vi "Get Test Info.vi"(7 "error in (no error)":errorcluster, 10 "Sequence Context In":T1) -> (0 "error out":errorcluster, 2 "Test Results":string[][](array[string]), 3 "Sequence Context out":T1)   [LabVIEW 2010]
uses:
  <vilib>/addons/TestStand/_TSLegacy.llb/LabVIEW Test - Sequence Context.ctl
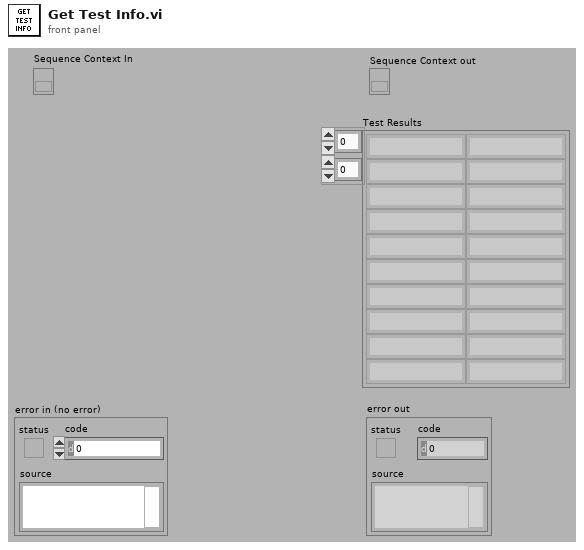
[diagram p1: front panel]
types:
  T1 = typedef "LabVIEW Test - Sequence Context.ctl" = refnum<k7>
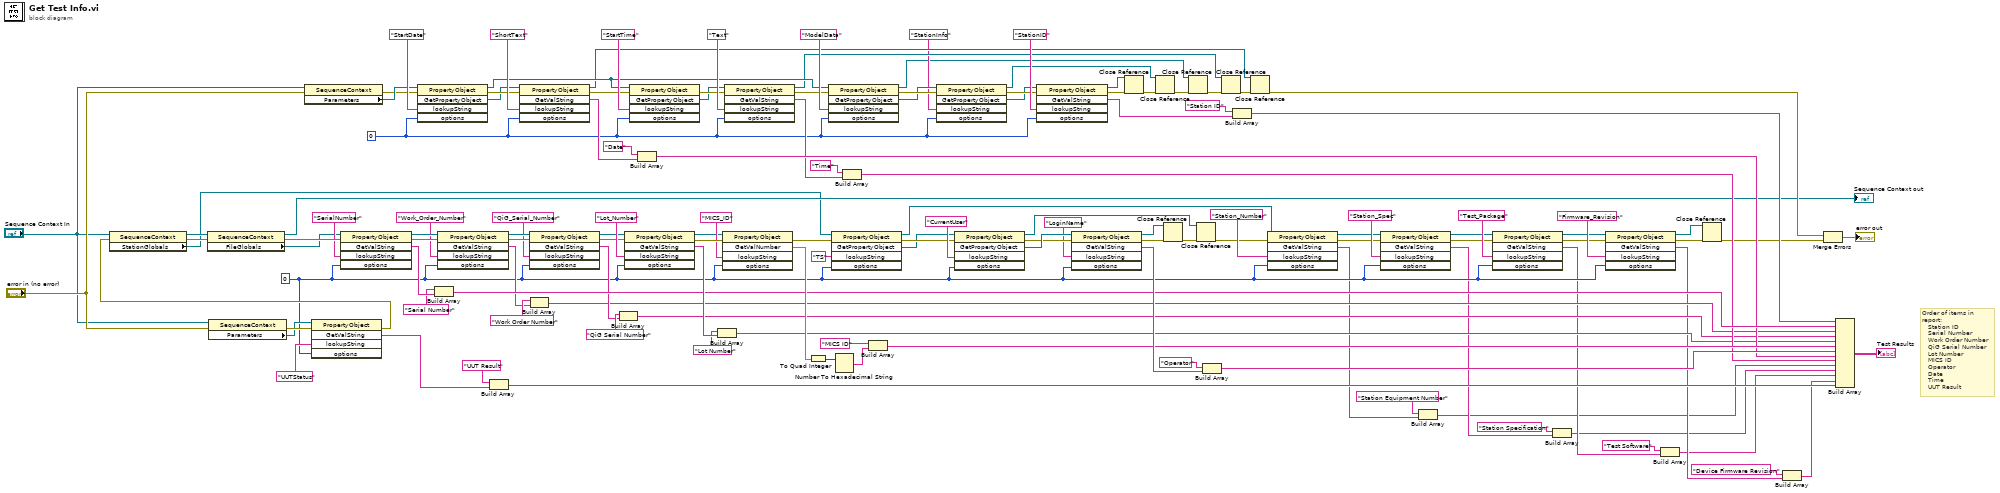
[diagram p0: block diagram]
diagram:
  w65 = 0
  w18 = 0
  # "Order of items in report:\n   Station ID\n   Serial Number\n   Work Order Number\n   QiG Serial Number\n   Lot Number\n   MICS ID\n   Operator\n   Date\n   Time\n   UUT Result"
  n1 = property class="SequenceContext"(reference="Sequence Context In", error in="error in (no error)") -> (error out=w37:errorcluster, "Parameters"=w36:refnum<k7>)  [unwired: 1 out]
  n2 = property class="SequenceContext"(reference="Sequence Context In", error in="error in (no error)") -> (error out=w95:errorcluster, "Parameters"=w100:refnum<k7>)  [unwired: 1 out]
  n3 = invoke class="PropertyObject" method="GetValString"(reference=w36, error in=w37, "lookupString"="UUTStatus", "options"=w18) -> (error out=w35:errorcluster, "GetValString"=w38:string)  [unwired: 1 in, 3 out]
  n4 = property class="SequenceContext"(reference="Sequence Context In", error in=w35) -> (reference out=w32:T1, error out=w34:errorcluster, "StationGlobals"=w31:refnum<k7>)
  n5 = property class="SequenceContext"(reference=w32, error in=w34) -> (reference out=→"Sequence Context out":T1, error out=w130:errorcluster, "FileGlobals"=w94:refnum<k7>)
  n6 = invoke class="PropertyObject" method="GetValString"(reference=w94, error in=w130, "lookupString"="SerialNumber", "options"=w18) -> (reference out=w55:refnum<k7>, error out=w54:errorcluster, "GetValString"=w124:string)  [unwired: 1 in, 2 out]
  n7 = invoke class="PropertyObject" method="GetPropertyObject"(reference=w100, error in=w95, "lookupString"="StartDate", "options"=w65) -> (reference out=w89:refnum<k7>, error out=w96:errorcluster, "GetPropertyObject"=w92:refnum<k7>)  [unwired: 1 in, 2 out]
  n8 = Build Array("Serial Number", w124) -> (w79:string[])
  n9 = invoke class="PropertyObject" method="GetValString"(reference=w55, error in=w54, "lookupString"="Work_Order_Number", "options"=w18) -> (reference out=w50:refnum<k7>, error out=w52:errorcluster, "GetValString"=w47:string)  [unwired: 1 in, 2 out]
  n10 = Build Array("UUT Result", w38) -> (w28:string[])
  n11 = invoke class="PropertyObject" method="GetValString"(reference=w92, error in=w96, "lookupString"="ShortText", "options"=w65) -> (reference out=w84:refnum<k7>, error out=w90:errorcluster, "GetValString"=w72:string)  [unwired: 1 in, 2 out]
  n12 = invoke class="PropertyObject" method="GetValString"(reference=w50, error in=w52, "lookupString"="QiG_Serial_Number", "options"=w18) -> (reference out=w46:refnum<k7>, error out=w51:errorcluster, "GetValString"=w44:string)  [unwired: 1 in, 2 out]
  n13 = Build Array("Work Order Number", w47) -> (w41:string[])
  n14 = Build Array("QiG Serial Number" ("lookupString"), w44) -> (w40:string[])
  n15 = invoke class="PropertyObject" method="GetValString"(reference=w46, error in=w51, "lookupString"="Lot_Number", "options"=w18) -> (reference out=w93:refnum<k7>, error out=w117:errorcluster, "GetValString"=w122:string)  [unwired: 1 in, 2 out]
  n16 = invoke class="PropertyObject" method="GetPropertyObject"(reference=w89, error in=w90, "lookupString"="StartTime", "options"=w65) -> (error out=w98:errorcluster, "GetPropertyObject"=w91:refnum<k7>)  [unwired: 1 in, 3 out]
  n17 = Build Array("Date" ("lookupString"), w72) -> (w74:string[])
  n18 = Build Array("Lot Number" ("lookupString"), w122) -> (w42:string[])
  n19 = invoke class="PropertyObject" method="GetValNumber"(reference=w93, error in=w117, "lookupString"="MICS_ID", "options"=w18) -> (error out=w115:errorcluster, "GetValNumber"=w112:dbl)  [unwired: 1 in, 3 out]
  n20 = invoke class="PropertyObject" method="GetValString"(reference=w91, error in=w98, "lookupString"="Text", "options"=w65) -> (reference out=w83:refnum<k7>, error out=w88:errorcluster, "GetValString"=w71:string)  [unwired: 1 in, 2 out]
  n21 = To Quad Integer(1:w112) -> (0:w113:i64)
  n22 = invoke class="PropertyObject" method="GetPropertyObject"(reference=w89, error in=w88, "lookupString"="ModelData", "options"=w65) -> (reference out=w62:refnum<k7>, error out=w69:errorcluster, "GetPropertyObject"=w67:refnum<k7>)  [unwired: 1 in, 2 out]
  n23 = invoke class="PropertyObject" method="GetPropertyObject"(reference=w31, error in=w115, "lookupString"="TS", "options"=w18) -> (reference out=w5:refnum<k7>, error out=w128:errorcluster, "GetPropertyObject"=w30:refnum<k7>)  [unwired: 1 in, 2 out]
  n24 = Number To Hexadecimal String(2:w113) -> (0:w114:string)  [unwired: 1 in]
  n25 = Build Array("Time" ("lookupString"), w71) -> (w73:string[])
  n26 = Build Array("MICS ID" ("lookupString"), w114) -> (w78:string[])
  n27 = invoke class="PropertyObject" method="GetPropertyObject"(reference=w67, error in=w69, "lookupString"="StationInfo", "options"=w65) -> (reference out=w57:refnum<k7>, error out=w68:errorcluster, "GetPropertyObject"=w64:refnum<k7>)  [unwired: 1 in, 2 out]
  n28 = invoke class="PropertyObject" method="GetPropertyObject"(reference=w30, error in=w128, "lookupString"="CurrentUser", "options"=w18) -> (reference out=w43:refnum<k7>, error out=w126:errorcluster, "GetPropertyObject"=w127:refnum<k7>)  [unwired: 1 in, 2 out]
  n29 = invoke class="PropertyObject" method="GetValString"(reference=w64, error in=w68, "lookupString"="StationID", "options"=w65) -> (reference out=w60:refnum<k7>, error out=w61:errorcluster, "GetValString"=w63:string)  [unwired: 1 in, 2 out]
  n30 = invoke class="PropertyObject" method="GetValString"(reference=w127, error in=w126, "lookupString"="LoginName", "options"=w18) -> (reference out=w106:refnum<k7>, error out=w107:errorcluster, "GetValString"=w120:string)  [unwired: 1 in, 2 out]
  n31 = Close Reference(reference=w60, error in (no error)=w61) -> (error out=w59:errorcluster)
  n32 = Close Reference(reference=w57, error in (no error)=w59) -> (error out=w58:errorcluster)
  n33 = Close Reference(reference=w106, error in (no error)=w107) -> (error out=w105:errorcluster)
  n34 = Close Reference(reference=w62, error in (no error)=w58) -> (error out=w87:errorcluster)
  n35 = Close Reference(reference=w43, error in (no error)=w105) -> (error out=w23:errorcluster)
  n36 = Build Array("Operator" ("lookupString"), w120) -> (w77:string[])
  n37 = Close Reference(reference=w83, error in (no error)=w87) -> (error out=w86:errorcluster)
  n38 = Build Array("Station ID" ("lookupString"), w63) -> (w80:string[])
  n39 = Close Reference(reference=w84, error in (no error)=w86) -> (error out=w85:errorcluster)
  n40 = invoke class="PropertyObject" method="GetValString"(reference=w5, error in=w23, "lookupString"="Station_Number", "options"=w18) -> (reference out=w4:refnum<k7>, error out=w22:errorcluster, "GetValString"=w13:string)  [unwired: 1 in, 2 out]
  n41 = invoke class="PropertyObject" method="GetValString"(reference=w4, error in=w22, "lookupString"="Station_Spec", "options"=w18) -> (reference out=w3:refnum<k7>, error out=w21:errorcluster, "GetValString"=w12:string)  [unwired: 1 in, 2 out]
  n42 = Build Array("Station Equipment Number" ("lookupString"), w13) -> (w9:string[])
  n43 = invoke class="PropertyObject" method="GetValString"(reference=w3, error in=w21, "lookupString"="Test_Package", "options"=w18) -> (reference out=w2:refnum<k7>, error out=w20:errorcluster, "GetValString"=w11:string)  [unwired: 1 in, 2 out]
  n44 = Build Array("Station Specification" ("lookupString"), w12) -> (w8:string[])
  n45 = invoke class="PropertyObject" method="GetValString"(reference=w2, error in=w20, "lookupString"="Firmware_Revision", "options"=w18) -> (reference out=w1:refnum<k7>, error out=w19:errorcluster, "GetValString"=w10:string)  [unwired: 1 in, 2 out]
  n46 = Build Array("Test Software" ("lookupString"), w11) -> (w7:string[])
  n47 = Close Reference(reference=w1, error in (no error)=w19) -> (error out=w29:errorcluster)
  n48 = Build Array("Device Firmware Revision" ("lookupString"), w10) -> (w6:string[])
  n49 = Merge Errors(w85, w29) -> (→"error out":errorcluster)
  n50 = Build Array(w80, w79, w41, w40, w42, w78, w77, w74, w73, w9, w8, w7, w6, w28) -> (→"Test Results":string[][])
